vi "ReadAndCheck.vi"(4 "GET":u8[](array[numeric])=[2, 80, 111, 0, 0, 0, 0, 0] format="%.0x", 6 "SET":u8[](array[numeric]) format="%x", 7 "ChanelIn":T2, 8 "errin":errorcluster, 10 "TA":u32 format="%.0x", 11 "SA":u32 format="%.0x") -> (0 "errout":errorcluster, 1 "Messout":T1, 2 "Identique":bool, 3 "trouvé":bool)   [LabVIEW 2020]
uses:
  C/Program Files (x86)/National Instruments/LabVIEW 2020/user.lib/PCAN Basic/Controls/Channel.ctl
  C/Program Files (x86)/National Instruments/LabVIEW 2020/user.lib/Alex_Peak_lib/PEAK_lib_ALEX.lvlib
  C/Program Files (x86)/National Instruments/LabVIEW 2020/user.lib/PCAN Basic/PCANBasic.lvlib
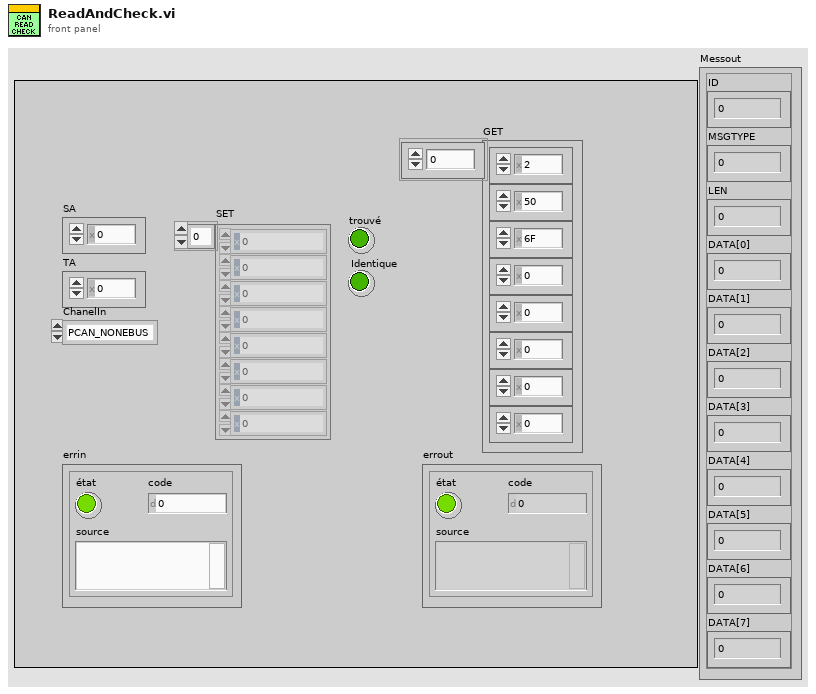
[diagram p1: front panel]
types:
  T1 = cluster{"ID":u32, "MSGTYPE":u8, "LEN":u8, "DATA[0]":u8, "DATA[1]":u8, "DATA[2]":u8, "DATA[3]":u8, "DATA[4]":u8, "DATA[5]":u8, "DATA[6]":u8, "DATA[7]":u8}
  T2 = typedef "PCANBasic.lvlib/Channel.ctl" = enum16{"PCAN_NONEBUS", "not used1", "not used2", "not used3", "not used4", "not used5", "not used6", "not used7", "not used8", "not used9", "not used10", "not used11", "not used12", "not used13", "not used14", "not used15", "not used16", "not used17", "not used18", "not used19", "not used20", "not used21", "not used22", "not used23", "not used24", "not used25", "not used26", "not used27", "not used28", "not used29", "not used30", "not used31", "not used32", "PCAN_ISABUS1", "PCAN_ISABUS2", "PCAN_ISABUS3", "PCAN_ISABUS4", "PCAN_ISABUS5", "PCAN_ISABUS6", "PCAN_ISABUS7", "PCAN_ISABUS8", "not used41", "not used42", "not used43", "not used44", "not used45", "not used46", "not used47", "not used48", "PCAN_DNGBUS1", "not used50", "not used51", "not used52", "not used53", "not used54", "not used55", "not used56", "not used57", "not used58", "not used59", "not used60", "not used61", "not used62", "not used63", "not used64", "PCAN_PCIBUS1", "PCAN_PCIBUS2", "PCAN_PCIBUS3", "PCAN_PCIBUS4", "PCAN_PCIBUS5", "PCAN_PCIBUS6", "PCAN_PCIBUS7", "PCAN_PCIBUS8", "not used73", "not used74", "not used75", "not used76", "not used77", "not used78", "not used79", "not used80", "PCAN_USBBUS1", "PCAN_USBBUS2", "PCAN_USBBUS3", "PCAN_USBBUS4", "PCAN_USBBUS5", "PCAN_USBBUS6", "PCAN_USBBUS7", "PCAN_USBBUS8", "Not used89", "Not used90", "Not used91", "Not used92", "Not used93", "Not used94", "Not used95", "Not used96", "PCAN_PCCBUS1", "PCAN_PCCBUS2"}
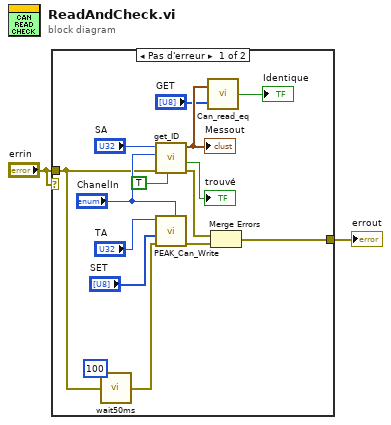
[diagram p0: block diagram]
diagram:
  n1 = case shown="Pas d'erreur" "errin" {
    tunnel: "errin" -> [w13 w18]
    tunnel: [w11 w18] -> w2
    frame No Error {
      n2 = call "wait50ms.vi"("attente (ms)"=u32 100, "errin"=w13) -> ("errout"=w12:errorcluster)  [unwired: 13 in]
      n3 = call "get_ID.vi"("Log?"=TRUE, "errin"=w13, "ChannelIn"="ChanelIn", "Identifier"="SA") -> ("errout"=w10:errorcluster, "trouvé"=→"trouvé":bool, "Messout"=w16:T1)  [unwired: 4 in, 1 out]
      "Messout" <- w16
      n4 = call "PEAK_Can_Write.vi"("CAN Handle"="ChanelIn", "errin"=w12, "CAN Data"="SET", "Identifier"="TA") -> ("errout"=w9:errorcluster)  [unwired: 7 in]
      n5 = call "Can_read_eq.vi"("TrameJeVeux"="GET", "MessIN"=w16) -> ("Identique"=→"Identique":bool)
      n6 = Merge Errors(w10, w9) -> (w11:errorcluster)
    }
    frame Error {
    }
  }
  "errout" <- w2
